vi "createCommand.vi"(8 "error in (no error)":errorcluster, 9 "Variant":variant, 10 "MonoCommand":T1=enum."getStatus", 11 "MonoClientCommunicator in":refnum<class "MonoClientCommunicator.lvclass">) -> (0 "error out":errorcluster, 2 "command":string, 3 "MonoClientCommunicator out":refnum<class "MonoClientCommunicator.lvclass">)   [LabVIEW 2016, in "MonoClientCommunicator.lvclass"]
uses:
  MonoClientCommunicator.lvclass
  Typedefs/MonoCommand.ctl
  Typedefs/wavelength.ctl
  Typedefs/slitWidth.ctl
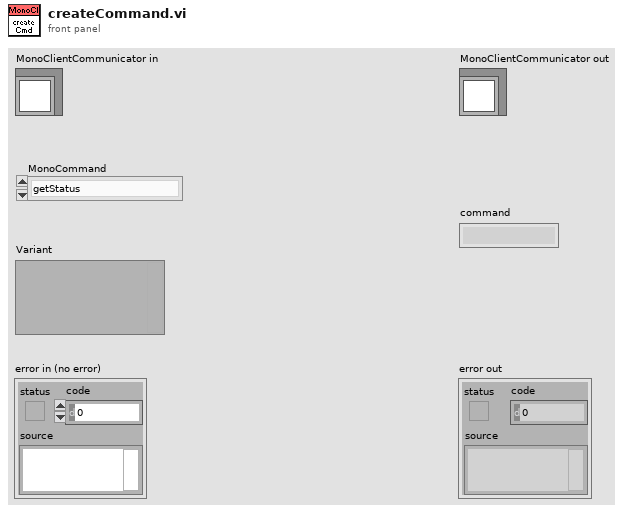
[diagram p1: front panel]
types:
  T1 = typedef "MonoCommand.ctl" = enum16{"getGrating", "getFrontEntranceSlitPosition", "getFrontExitSlitPosition", "getWavelength", "setWavelength", "setGrating", "setFrontEntranceSlitPosition", "setFrontExitSlitPosition", "calibrateWavelength", "getStatus", "Unknown", "reset"}
  T2 = typedef "wavelength.ctl" = dbl
  T3 = typedef "slitWidth.ctl" = dbl
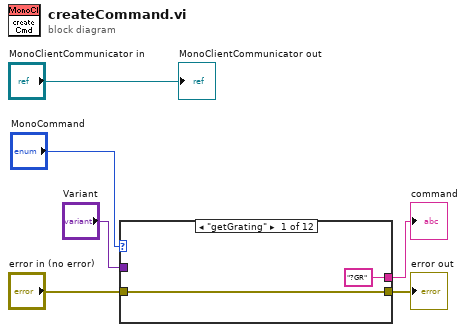
[diagram p0: block diagram]
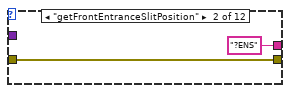
[diagram p2: hidden frame]
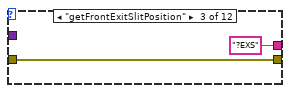
[diagram p3: hidden frame]
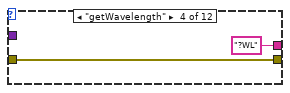
[diagram p4: hidden frame]
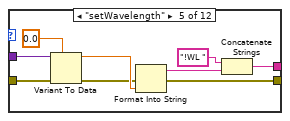
[diagram p5: hidden frame]
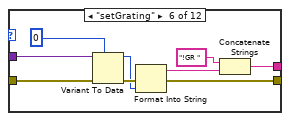
[diagram p6: hidden frame]
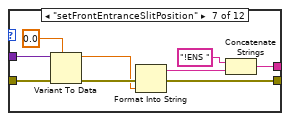
[diagram p7: hidden frame]
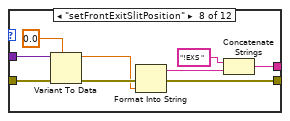
[diagram p8: hidden frame]
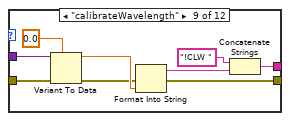
[diagram p9: hidden frame]
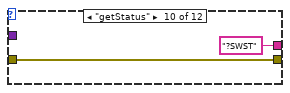
[diagram p10: hidden frame]
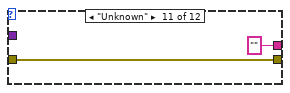
[diagram p11: hidden frame]
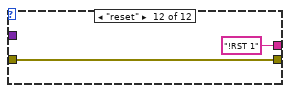
[diagram p12: hidden frame]
diagram:
  n1 = case shown="\"getGrating\"" "MonoCommand" {
    tunnel: "Variant" -> [_ _ _ _ w22 w32 w34 w44 w52 _ _ _]
    tunnel: ["?GR" "?ENS" "?EXS" "?WL" w15 w27 w40 w49 w57 "?SWST" "" "!RST 1"] -> w3
    tunnel: "error in (no error)" -> [w7 w9 w11 w13 w21 w31 w38 w45 w53 w61 w63 w64]
    tunnel: [w7 w9 w11 w13 w16 w30 w39 w48 w55 w61 w63 w64] -> w1
    frame "getGrating" {
    }
    frame "getFrontEntranceSlitPosition" {
    }
    frame "getFrontExitSlitPosition" {
    }
    frame "getWavelength" {
    }
    frame "setWavelength" {
      n2 = Variant To Data(error in=w21, type=T2 0.0 ("wavelength"), Variant=w22) -> (data=w19:T2, error out=w17:errorcluster)
      n3 = Format Into String(error in=w17, w19) -> (resulting string=w18:string, error out=w16:errorcluster)  [unwired: 2 in]
      n4 = Concatenate Strings("!WL ", w18) -> (w15:string)
    }
    frame "setGrating" {
      n5 = Variant To Data(error in=w31, type=u16 0, Variant=w32) -> (data=w28:u16, error out=w29:errorcluster)
      n6 = Format Into String(error in=w29, w28) -> (resulting string=w26:string, error out=w30:errorcluster)  [unwired: 2 in]
      n7 = Concatenate Strings("!GR " ("string"), w26) -> (w27:string)
    }
    frame "setFrontEntranceSlitPosition" {
      n8 = Variant To Data(error in=w38, type=T3 0.0 ("position"), Variant=w34) -> (data=w36:T3, error out=w37:errorcluster)
      n9 = Format Into String(error in=w37, w36) -> (resulting string=w35:string, error out=w39:errorcluster)  [unwired: 2 in]
      n10 = Concatenate Strings("!ENS " ("string"), w35) -> (w40:string)
    }
    frame "setFrontExitSlitPosition" {
      n11 = Variant To Data(error in=w45, type=T3 0.0 ("position"), Variant=w44) -> (data=w43:T3, error out=w46:errorcluster)
      n12 = Format Into String(error in=w46, w43) -> (resulting string=w47:string, error out=w48:errorcluster)  [unwired: 2 in]
      n13 = Concatenate Strings("!EXS " ("string"), w47) -> (w49:string)
    }
    frame "calibrateWavelength" {
      n14 = Variant To Data(error in=w53, type=T2 0.0 ("wavelength"), Variant=w52) -> (data=w59:T2, error out=w54:errorcluster)
      n15 = Format Into String(error in=w54, w59) -> (resulting string=w56:string, error out=w55:errorcluster)  [unwired: 2 in]
      n16 = Concatenate Strings("!CLW " ("string"), w56) -> (w57:string)
    }
    frame "getStatus" {
    }
    frame "Unknown" {
    }
    frame "reset" {
    }
  }
  "error out" <- w1
  "command" <- w3
  "MonoClientCommunicator out" <- "MonoClientCommunicator in"
